vi "PrepareChannels_DigitalOnly.vi"(1 "DO Physical channels":tag="pciDAQ/port0/line1:2") -> (9 "DO task out":refnum<k21>, 10 "DO error out":errorcluster)   [LabVIEW 2017]
uses:
  <vilib>/DAQmx/create/channels.llb/DAQmx Create Channel (DO-Digital Output).vi
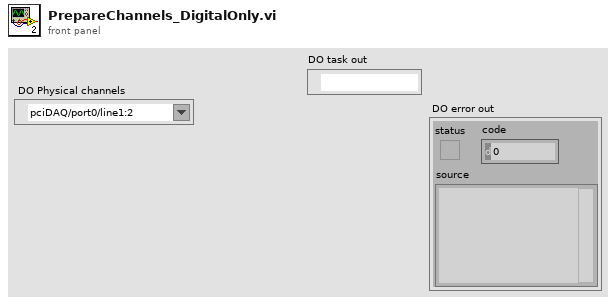
[diagram p1: front panel]
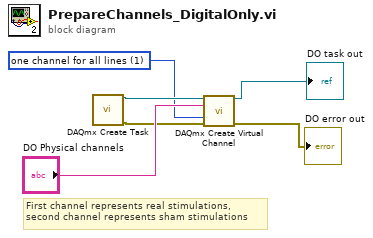
[diagram p0: block diagram]
diagram:
  w1 = 1 items=["one channel for each line", "one channel for all lines"] ("line grouping")
  # "First channel represents real stimulations,\nsecond channel represents sham stimulations"
  n1 = call <vilib>:"DAQmx Create Task.vi"() -> ("task out"=w5:refnum<k21>, "error out"=w4:errorcluster)  [unwired: 14 in]
  n2 = call-poly <vilib>:"DAQmx Create Virtual Channel.vi"("task in"=w5, "lines"="DO Physical channels", "line grouping"=w1, "error in"=w4) -> ("task out"=→"DO task out":refnum<k21>, "error out"=→"DO error out":errorcluster)  [unwired: 10 in]
